vi "AnalysePacket.vi"(6 "AdjustPacketSize":bool, 8 "error in":errorcluster, 9 "Offset":i32, 11 "Data":bool[](array[boolean])) -> (0 "error out":errorcluster, 1 "OffsetOut":i32, 3 "Result":u64)   [LabVIEW 2020, in "2021_16.lvclass"]
uses:
  2021_16.lvclass
  16_Helper_class/16_Helper.lvclass
panel:
  out "Array":u64[](array[numeric])
  out "Total Length Of Sub-Packets Or\nNumber Of Sub-Packets":u32
  out "Type":u32
  out "Version":u32
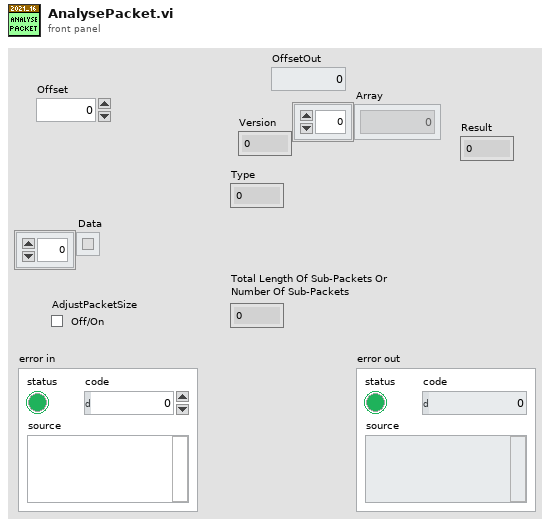
[diagram p1: front panel]
types:
  T1 = enum16{"sum", "Product", "Minimum", "Maximum", "Number", "Greater Than", "Less Than", "Equal To"}
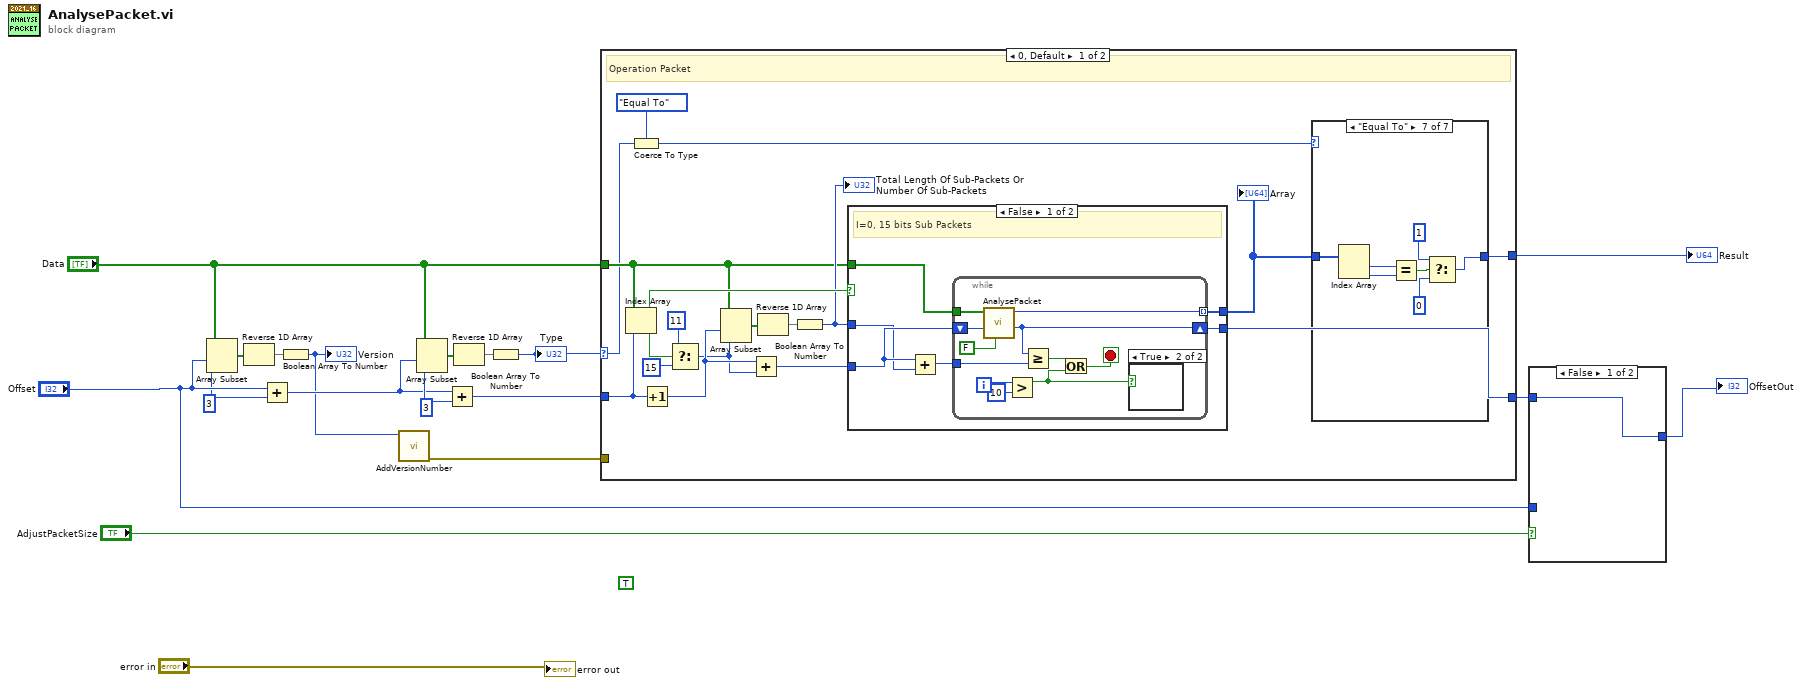
[diagram p0: block diagram]
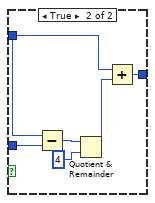
[diagram p2: hidden frame]
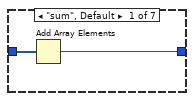
[diagram p3: hidden frame]
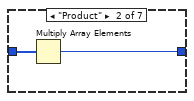
[diagram p4: hidden frame]
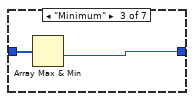
[diagram p5: hidden frame]
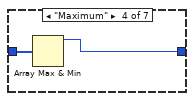
[diagram p6: hidden frame]
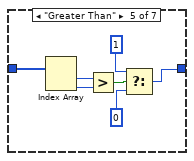
[diagram p7: hidden frame]
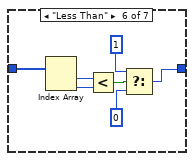
[diagram p8: hidden frame]
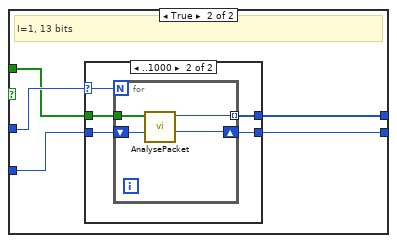
[diagram p10: hidden frame]
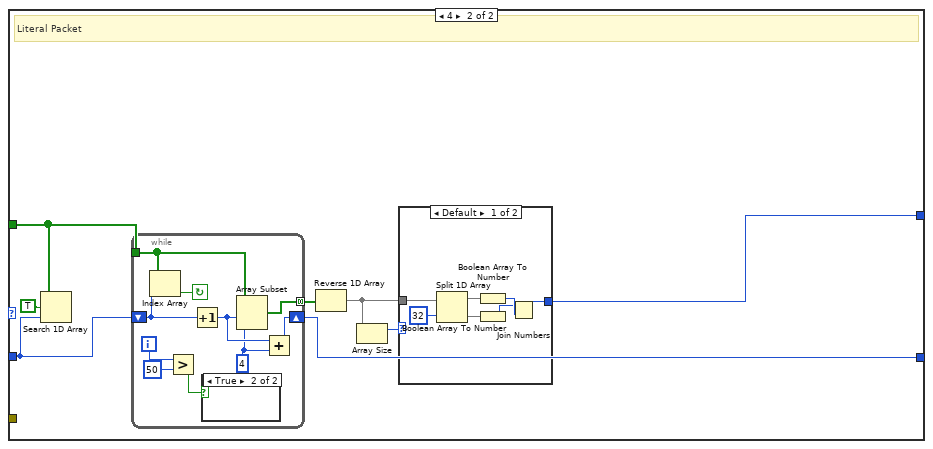
[diagram p12: hidden frame]
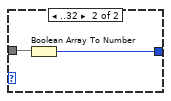
[diagram p13: hidden frame]
diagram:
  (unwired) TRUE
  w9 = 3 ("length")
  w12 = 3 ("length")
  n1 = Array Subset(array="Data", index="Offset", length=w12) -> (w14:bool[])
  n2 = Reverse 1D Array(array=w14) -> (reversed array=w13:bool[])
  n3 = Add(x="Offset", y=w12) -> (x+y=w8:i32)
  n4 = Boolean Array To Number(Boolean array=w13) -> (number=w5:u32)
  "Version" <- w5
  n5 = call "AddVersionNumber.vi"("VersionNumber"=w5) -> ("Error Out"=w1:errorcluster)  [unwired: 10 in]
  n6 = Array Subset(array="Data", index=w8, length=w9) -> (w10:bool[])
  n7 = Add(x=w8, y=w9) -> (x+y=w7:i32)
  n8 = Reverse 1D Array(array=w10) -> (reversed array=w11:bool[])
  n9 = Boolean Array To Number(Boolean array=w11) -> (number=w6:u32)
  "Type" <- w6
  n10 = case shown="0, Default" w6 {
    selector: w6 -> [w22 _]
    tunnel: "Data" -> [w26 w103]
    tunnel: w7 -> [w35 w98]
    tunnel: [w19 w97] -> w16
    tunnel: [w24 w99] -> w4
    tunnel: w1 -> [_ _]
    frame 0, Default {
      # "Operation Packet"
      n11 = Index Array(array=w26, index=w35) -> (element=w28:bool)
      n12 = Coerce To Type(0:w22, 1:T1."Equal To") -> (2:w21:T1)
      n13 = Increment(x=w35) -> (x+1=w34:i32)
      n14 = Select(t=11 ("length"), s=w28, f=15 ("length")) -> (s? t:f=w29:i32)
      n15 = Array Subset(array=w26, index=w34, length=w29) -> (w33:bool[])
      n16 = Add(x=w34, y=w29) -> (x+y=w25:i32)
      n17 = Reverse 1D Array(array=w33) -> (reversed array=w32:bool[])
      n18 = Boolean Array To Number(Boolean array=w32) -> (number=w27:u32)
      "Total Length Of Sub-Packets Or\nNumber Of Sub-Packets" <- w27
      n19 = case shown="False" w28 {
        tunnel: w27 -> [w67 w86]
        tunnel: w26 -> [w69 w85]
        tunnel: w25 -> [w68 w84]
        tunnel: [w70 w83] -> w24
        tunnel: [w65 w82] -> w20
        frame False {
          # "I=0, 15 bits Sub Packets"
          n20 = Add(x=w68, y=w67) -> (x+y=w66:u32)
          n21 = while {
            tunnel: w69 -> [w81]
            tunnel: w66 -> [w80]
            shift-right: [w78] -> w70
            shift-left: w68 -> [w79]
            tunnel: [w77] -> w65 mode=indexing
            i -> [w75]
            stop <- w71 stop-if-true
            n22 = call "AnalysePacket.vi"("AdjustPacketSize"=FALSE, "Offset"=w79, "Data"=w81) -> ("OffsetOut"=w78:i32, "Result"=w77:u64)  [unwired: 6 in, 1 out]
            n23 = Greater?(x=w75, y=10) -> (0:w72:bool)
            n24 = Greater Or Equal?(x=w78, y=w80) -> (x >= y?=w73:bool)
            n25 = Or(x=w73, y=w72) -> (x .or. y?=w71:bool)
            n26 = case shown="True" w72 {
              frame False {
              }
              frame True {
              }
            }
          }
        }
        frame True {
          # "I=1, 13 bits"
          n27 = case shown="..1000" w86 {
            selector: w86 -> [_ w92]
            tunnel: w85 -> [_ w91]
            tunnel: w84 -> [w87 w90]
            tunnel: [_ w89] -> w82
            tunnel: [w87 w88] -> w83
            frame Default {
            }
            frame ..1000 {
              n28 = for {
                N: w92 -> [_]
                tunnel: w91 -> [w96]
                shift-right: [w94] -> w88
                shift-left: w90 -> [w95]
                tunnel: [w93] -> w89 mode=indexing
                n29 = call "AnalysePacket.vi"("Offset"=w95, "Data"=w96) -> ("OffsetOut"=w94:i32, "Result"=w93:u64)  [unwired: 7 in, 1 out]
              }
            }
          }
        }
      }
      "Array" <- w20
      n30 = case shown="\"Equal To\"" w21 {
        tunnel: w20 -> [w37 w39 w41 w43 w50 w57 w64]
        tunnel: [w36 w38 w40 w42 w44 w51 w58] -> w19
        frame "sum", Default {
          n31 = Add Array Elements(numeric array=w37) -> (sum=w36:u64)
        }
        frame "Product" {
          n32 = Multiply Array Elements(1:w39) -> (0:w38:u64)
        }
        frame "Minimum" {
          n33 = Array Max & Min(array=w41) -> (min value=w40:u64)  [unwired: 3 out]
        }
        frame "Maximum" {
          n34 = Array Max & Min(array=w43) -> (max value=w42:u64)  [unwired: 3 out]
        }
        frame "Greater Than" {
          n35 = Index Array(array=w50) -> (element #1=w49:u64, element #2=w48:u64)  [unwired: 2 in]
          n36 = Greater?(x=w49, y=w48) -> (0:w47:bool)
          n37 = Select(t=u64 1, s=w47, f=u64 0) -> (s? t:f=w44:u64)
        }
        frame "Less Than" {
          n38 = Index Array(array=w57) -> (element #1=w56:u64, element #2=w55:u64)  [unwired: 2 in]
          n39 = Less?(x=w56, y=w55) -> (x < y?=w54:bool)
          n40 = Select(t=u64 1, s=w54, f=u64 0) -> (s? t:f=w51:u64)
        }
        frame "Equal To" {
          n41 = Index Array(array=w64) -> (element #1=w63:u64, element #2=w62:u64)  [unwired: 2 in]
          n42 = Equal?(x=w63, y=w62) -> (x = y?=w61:bool)
          n43 = Select(t=u64 1, s=w61, f=u64 0) -> (s? t:f=w58:u64)
        }
      }
    }
    frame 4 {
      # "Literal Packet"
      n44 = Search 1D Array(1D array=w103, element=TRUE, start index (0)=w98) -> ()  [unwired: 1 out]
      n45 = while {
        tunnel: w103 -> [w122]
        shift-right: [w118] -> w99
        shift-left: w98 -> [w123]
        tunnel: [w117] -> w102 mode=concatenating
        i -> [w116]
        stop <- w121 continue-if-true
        w119 = 4 ("length")
        n46 = Index Array(array=w122, index=w123) -> (element=w121:bool)
        n47 = Greater?(x=w116, y=50) -> (0:w114:bool)
        n48 = Increment(x=w123) -> (x+1=w120:i32)
        n49 = case shown="True" w114 {
          frame False {
          }
          frame True {
          }
        }
        n50 = Array Subset(array=w122, index=w120, length=w119) -> (w117:bool[])
        n51 = Add(x=w120, y=w119) -> (x+y=w118:i32)
      }
      n52 = Reverse 1D Array(array=w102) -> (reversed array=w101:bool[])
      n53 = Array Size(array=w101) -> (size(s)=w100:i32)
      n54 = case shown="Default" w100 {
        tunnel: [w105 w113] -> w97
        tunnel: w101 -> [w111 w112]
        frame Default {
          n55 = Split 1D Array(array=w111, index=32) -> (first subarray=w109:bool[], second subarray=w108:bool[])
          n56 = Boolean Array To Number(Boolean array=w109) -> (number=w107:u32)
          n57 = Boolean Array To Number(Boolean array=w108) -> (number=w106:u32)
          n58 = Join Numbers(hi=w106, lo=w107) -> ((hi.lo)=w105:u64)
        }
        frame ..32 {
          n59 = Boolean Array To Number(Boolean array=w112) -> (number=w113:u32)
        }
      }
    }
  }
  "Result" <- w16
  n60 = case shown="False" "AdjustPacketSize" {
    tunnel: "Offset" -> [_ w130]
    tunnel: w4 -> [w124 w126]
    tunnel: [w124 w125] -> w3
    frame False {
    }
    frame True {
      n61 = Subtract(x=w126, y=w130) -> (x-y=w129:i32)
      n62 = Quotient & Remainder(x=w129, y=4) -> (x-y*floor(x/y)=w127:i32)  [unwired: 1 out]
      n63 = Add(x=w126, y=w127) -> (x+y=w125:i32)
    }
  }
  "OffsetOut" <- w3
  "error out" <- "error in"
